vi "Calculate Mean by Derivatives.vi"(4 "Waveform":waveform(dbl)) -> (1 "Waveform Mean":waveform(dbl))   [LabVIEW 2013]
uses:
  <vilib>/Analysis/NI_AALPro.lvlib
  <vilib>/gmath/NI_Gmath.lvlib
panel:
  out "d2y/dt2":waveform(dbl)(graph)
  out "dy/dt":waveform(dbl)(graph)
  out "Signal":waveform(dbl)(graph)
  out "Minima":waveform(dbl)(graph)
  out "Maxima":waveform(dbl)(graph)
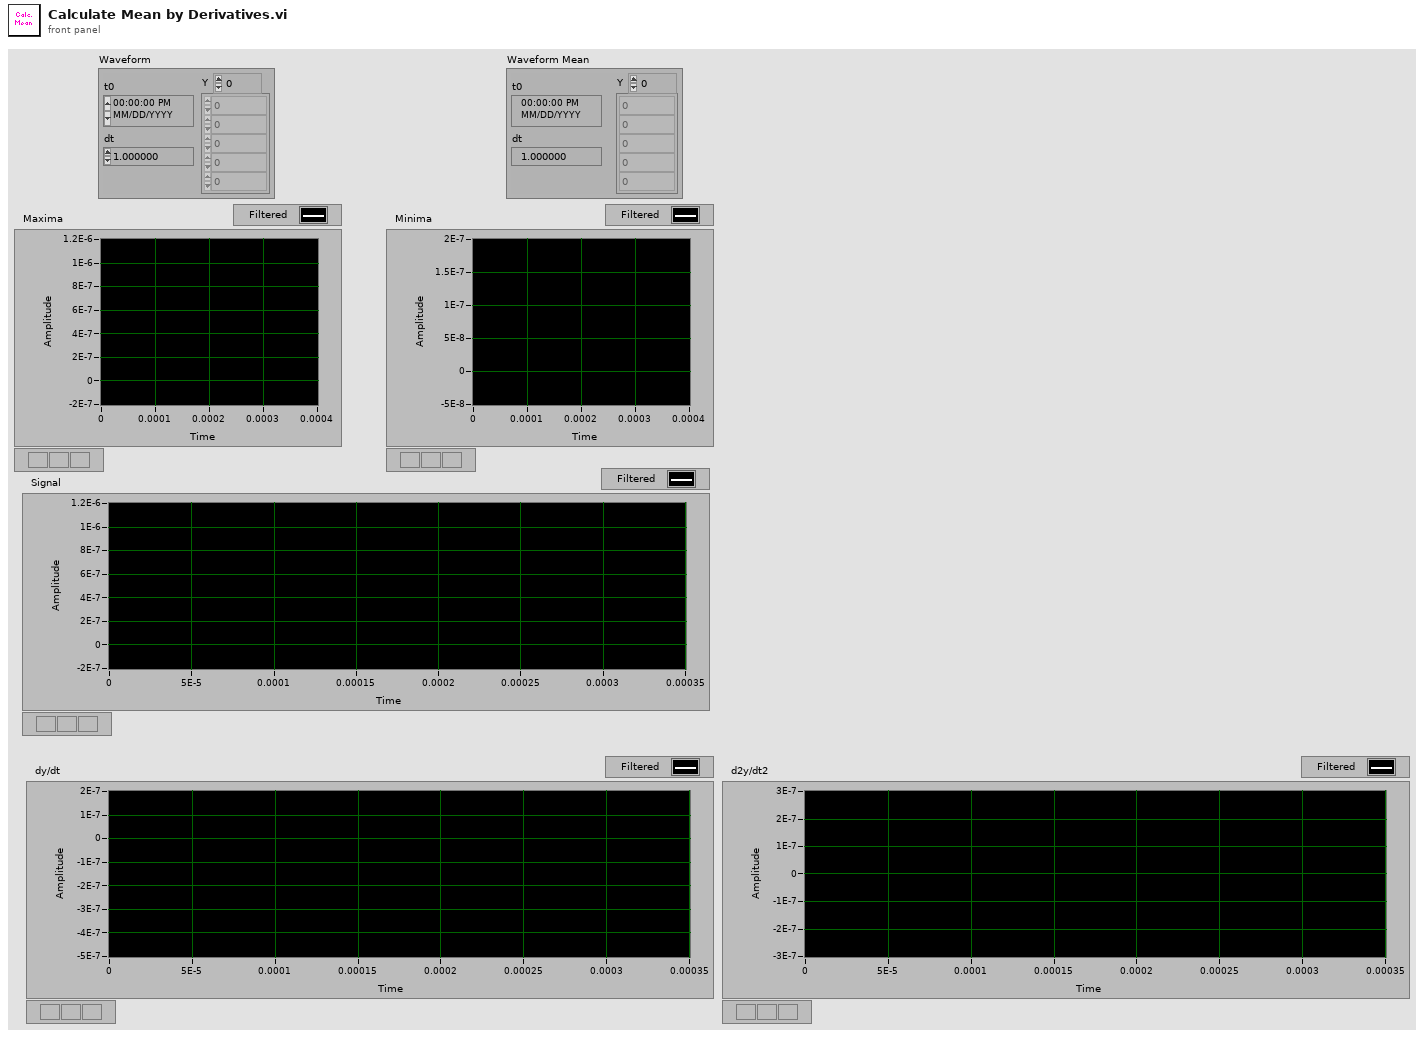
[diagram p1: front panel]
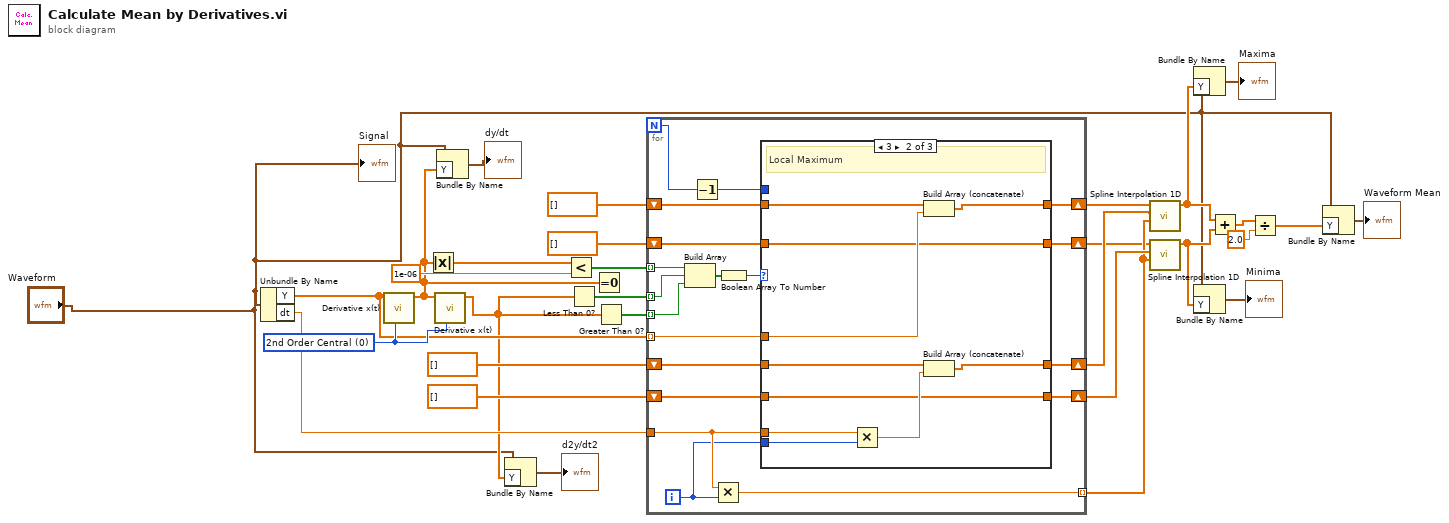
[diagram p0: block diagram]
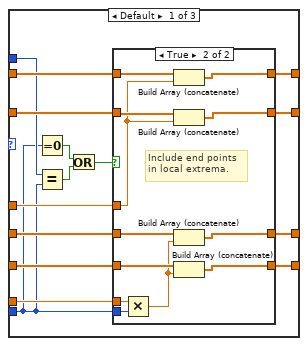
[diagram p2: hidden frame]
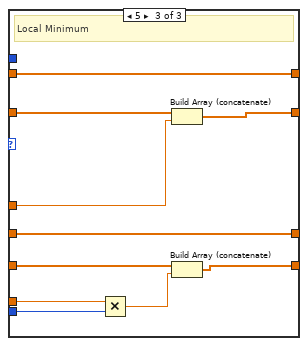
[diagram p4: hidden frame]
diagram:
  w17 = u16 0 items=["2nd Order Central", "4th Order Central", "Forward", "Backward"] ("method")
  n1 = Unbundle By Name("Waveform") -> ("Y"=w8:dbl[], "dt"=w9:dbl)
  n2 = call <vilib>:"Derivative x(t).vi"("method"=w17, "X"=w8) -> ("dX/dt"=w11:dbl[])  [unwired: 8 in, 1 out]
  n3 = Absolute Value(x=w11) -> (abs(x)=w12:dbl[])
  n4 = call <vilib>:"Derivative x(t).vi"("method"=w17, "X"=w11) -> ("dX/dt"=w3:dbl[])  [unwired: 8 in, 1 out]
  n5 = Bundle By Name(cluster="Waveform", "Y"=w11) -> (→"dy/dt":waveform(dbl))
  n6 = Bundle By Name(cluster="Waveform", "Y"=w3) -> (→"d2y/dt2":waveform(dbl))
  n7 = Less?(x=w12, y=1e-06 ("dt")) -> (x < y?=w13:bool[])
  n8 = Less Than 0?(x=w3) -> (x < 0?=w30:bool[])
  n9 = Equal To 0?(x=w11) -> ()  [unwired: 1 out]
  n10 = Greater Than 0?(x=w3) -> (x > 0?=w18:bool[])
  n11 = for {
    N -> [w32]
    tunnel: w13 -> [w49] mode=indexing
    tunnel: w8 -> [w45] mode=indexing
    tunnel: w9 -> [w36]
    tunnel: w30 -> [w48] mode=indexing
    shift-right: [w40] -> w15
    shift-left: dbl[] [] -> [w44]
    shift-right: [w38] -> w14
    shift-left: dbl[] [] -> [w43]
    shift-right: [w39] -> w25
    shift-left: dbl[] [] -> [w42]
    shift-right: [w37] -> w24
    shift-left: dbl[] [] -> [w41]
    tunnel: [w34] -> w23 mode=indexing
    tunnel: w18 -> [w33] mode=indexing
    i -> [w35]
    n12 = Build Array(w49, w48, w33) -> (w47:bool[])
    n13 = Decrement(x=w32) -> (x-1=w31:i32)
    n14 = Multiply(x=w36, y=w35) -> (x*y=w34:dbl)
    n15 = Boolean Array To Number(Boolean array=w47) -> (number=w46:u32)
    n16 = case shown="3" w46 {
      tunnel: w45 -> [w59 w89 w100]
      tunnel: w36 -> [w60 w86 w98]
      tunnel: w35 -> [w53 w87 w99]
      tunnel: w44 -> [w64 w90 w94]
      tunnel: w43 -> [w63 w82 w96]
      tunnel: w42 -> [w62 w88 w93]
      tunnel: w41 -> [w61 w81 w95]
      tunnel: [w58 w84 w94] -> w40
      tunnel: [w56 w83 w93] -> w39
      tunnel: [w57 w82 w92] -> w38
      tunnel: [w55 w81 w91] -> w37
      tunnel: w31 -> [w54 _ _]
      frame Default {
        n17 = Equal To 0?(x=w53) -> (x = 0?=w52:bool)
        n18 = Equal?(x=w54, y=w53) -> (x = y?=w51:bool)
        n19 = Or(x=w52, y=w51) -> (x .or. y?=w50:bool)
        n20 = case shown="True" w50 {
          tunnel: w64 -> [w68 w80]
          tunnel: w63 -> [w67 w75]
          tunnel: w62 -> [w66 w78]
          tunnel: w61 -> [w65 w71]
          tunnel: w60 -> [_ w77]
          tunnel: w59 -> [_ w74]
          tunnel: [w68 w79] -> w58
          tunnel: [w67 w73] -> w57
          tunnel: [w66 w72] -> w56
          tunnel: [w65 w69] -> w55
          tunnel: w53 -> [_ w76]
          frame False {
          }
          frame True {
            # "Include end points\nin local extrema."
            n21 = Multiply(x=w77, y=w76) -> (x*y=w70:dbl)
            n22 = Build Array (concatenate)(w80, w74) -> (w79:dbl[])
            n23 = Build Array (concatenate)(w75, w74) -> (w73:dbl[])
            n24 = Build Array (concatenate)(w78, w70) -> (w72:dbl[])
            n25 = Build Array (concatenate)(w71, w70) -> (w69:dbl[])
          }
        }
      }
      frame 3 {
        # "Local Maximum"
        n26 = Multiply(x=w86, y=w87) -> (x*y=w85:dbl)
        n27 = Build Array (concatenate)(w90, w89) -> (w84:dbl[])
        n28 = Build Array (concatenate)(w88, w85) -> (w83:dbl[])
      }
      frame 5 {
        # "Local Minimum"
        n29 = Multiply(x=w98, y=w99) -> (x*y=w97:dbl)
        n30 = Build Array (concatenate)(w96, w100) -> (w92:dbl[])
        n31 = Build Array (concatenate)(w95, w97) -> (w91:dbl[])
      }
    }
  }
  n32 = call <vilib>:"Spline Interpolation 1D.vi"("xi"=w23, "X"=w25, "Y"=w15) -> ("yi"=w7:dbl[])  [unwired: 6 in, 2 out]
  n33 = call <vilib>:"Spline Interpolation 1D.vi"("xi"=w23, "X"=w24, "Y"=w14) -> ("yi"=w5:dbl[])  [unwired: 6 in, 2 out]
  n34 = Bundle By Name(cluster="Waveform", "Y"=w7) -> (→"Maxima":waveform(dbl))
  n35 = Bundle By Name(cluster="Waveform", "Y"=w5) -> (→"Minima":waveform(dbl))
  n36 = Add(x=w7, y=w5) -> (x+y=w22:dbl[])
  n37 = Divide(x=w22, y=2.0) -> (x/y=w20:dbl[])
  n38 = Bundle By Name(cluster="Waveform", "Y"=w20) -> (→"Waveform Mean":waveform(dbl))
  "Signal" <- "Waveform"
